vi "H5Tget_super.vi"(6 "error in (no error)":errorcluster, 9 "HDF5 Type Ref":T1) -> (0 "error out":errorcluster, 2 "HDF5 Super Type Ref":T1, 3 "HDF5 Type Ref out":T1)   [LabVIEW 2017]
doc: "Returns the base datatype from which a datatype is derived."
uses:
  <vilib>/UPVI/lvhdf5/library.llb/HDF5 Ref.ctl
  <vilib>/UPVI/lvhdf5/hdf5.dll
panel:
  # "LVHDF5 Toolkit\nCopyright (c) 2005-2013 by Jason D. Sommerville\nCopyright (c) 2014 by UPVI, LLC.\n\nThis use and distribution of this file is governed by the terms found in \nLICENSE.txt distributed with this toolkit and installed at\n <user.lib>\\_lvhdf5\\LICENSE.txt"
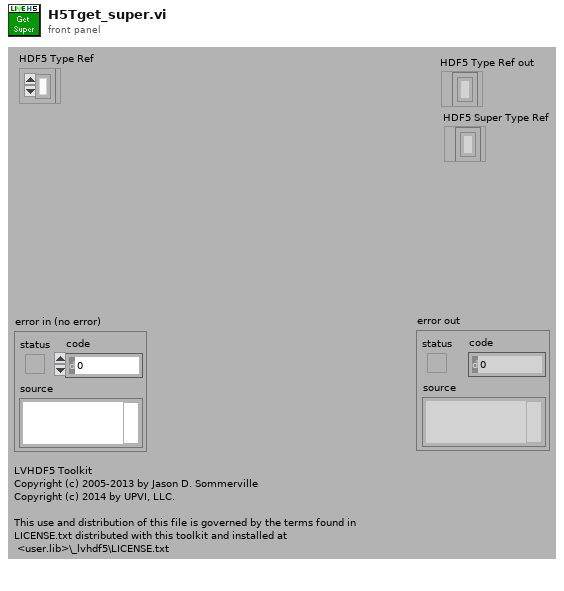
[diagram p1: front panel]
types:
  T1 = typedef "HDF5 Ref.ctl" = refnum<k1>
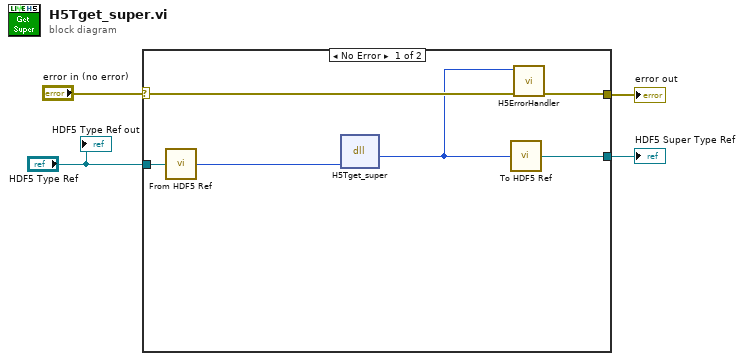
[diagram p0: block diagram]
diagram:
  n1 = case shown="No Error" "error in (no error)" {
    selector: "error in (no error)" -> [w10 w11]
    tunnel: [w9 w11] -> w3
    tunnel: "HDF5 Type Ref" -> [w8 _]
    tunnel: [w5 _] -> w1
    frame No Error {
      n2 = call <vilib>:"From HDF5 Ref.vi"("HDF5 Ref"=w8) -> ("I32"=w7:i32)
      n3 = dll-call lib="C:/Program Files/National Instruments/LabVIEW 2017/vi.lib/UPVI/lvhdf5/hdf5.dll" fn="H5Tget_super"("loc_id"=w7) -> ("return type"=w6:i32)  [unwired: 4 in, 2 out]
      n4 = call <vilib>:"To HDF5 Ref.vi"("I32"=w6) -> ("HDF5 Ref"=w5:T1)
      n5 = call <vilib>:"H5ErrorHandler.vi"("error in (no error)"=w10, "herr_t"=w6) -> ("error out"=w9:errorcluster)  [unwired: 3 in, 4 out]
    }
    frame Error {
    }
  }
  "error out" <- w3
  "HDF5 Super Type Ref" <- w1
  "HDF5 Type Ref out" <- "HDF5 Type Ref"
